vi "ProstateGetData.vi"() -> ()   [LabVIEW 2022 SP3]
uses:
  <instrlib>/vi.lib/Platform/portaccess.llb/Out Port8.vi
  <vilib>/DAQmx/create/channels.llb/DAQmx Create Channel (CO-Pulse Generation-Time).vi
  <resource>/objmgr/daqmx.rc
  <vilib>/DAQmx/configure/trigger.llb/DAQmx Start Trigger (Digital Edge).vi
  ScanningControl/Motion Controllers/-MotionRoutines/MotionGlobals.vi
  ScanningControl/Digitizers/-DigitizerRoutines/Digitizer.ctl
  ViewData/-ReadEye/ScaleMethod.ctl
  ScanningControl/Digitizers/-DigitizerRoutines/DigitizerID.ctl
  ScanningControl/Digitizers/-DigitizerRoutines/DigitizerSettings.ctl
  ScanningControl/Digitizers/-DigitizerRoutines/DigConfig.ctl
  C:/Windows/System32/ADQAPI_dotNet_helper.dll
panel:
  out "Digitizer Settings":T1={"Digitizer delay (us) "=0.0, "rf points per line"=2048, "lines per plane"=128, "Samp Rate (Hz)"=100000000.0, "Additional dig delay (us)"=0.0, "Voltage Scale"=0.4, "Pre-Looks"=0, "Offset delay (us)"=0.0, "bits A/D"=8, "Avg Num"=1, "DigTimeOut"=5.0, "Rel Dig Delay"=0.0, "Dig Ch"=0, "LeCroyCluster"={"LeCroy Channels"=[TRUE, FALSE, FALSE, FALSE], "LC read pt offset"=0.0, "Sweep Avg"=FALSE}, "Main Digitizer"=enum."NI Digitizer", "Dig Config"=enum."Single channel", "Digitizer ID Cluster"={"Acqiris/Alazar/SP ID"=[], "NI Instr Handles"=[], "LeCroy VISA"="", "GaGe Handle"={"Handle"=0, "Sample size"=0, "Resolution"=0, "Offset"=0, "Channels"=0, "Boards"=0}, "ATS Ref"="ATS9350", "Acqiris Address"=["PCI::INSTR0"], "ADQRef"=refnum, "adq_cu_ptr"=refnum}, "Trigger Settings"={"Trig Source"=1, "Trig Coupling"=0, "Trig Slope"=0, "Level (mV)"=1500.0}, "Bulk Acq"=FALSE, "Bulk Start Indexes"=[], "Data Ref RF"=refnum, "NI ID/Channel"=[], "Total Dig CH"=5, "Xtra Ann Trig delay (us)"=10.0, "Fix Z Delay?"=FALSE, "One Way Transmission?"=FALSE, "Data Ref Log"=refnum} {"Trigger Settings"."Trig Slope" items=["Positive", "Negative"]; "Trigger Settings"."Level (mV)" format="%.2f"; "Trigger Settings"."Trig Coupling" items=["DC 1 MOhm", "AC 1 MOhm", "DC 50 Ohm", "AC 50 Ohm"]; "Trigger Settings"."Trig Source" items=["Chan 1", "External"]; "Rel Dig Delay" format="%.2f"; "DigTimeOut" format="%.2f"; "Avg Num" min=1; "Offset delay (us)" format="%.2f"; "Additional dig delay (us)" format="%.2f"; "Digitizer delay (us)" format="%.2f"}
  in  "Digitizer Settings":T1={"Digitizer delay (us) "=0.0, "rf points per line"=2048, "lines per plane"=128, "Samp Rate (Hz)"=100000000.0, "Additional dig delay (us)"=0.0, "Voltage Scale"=0.4, "Pre-Looks"=0, "Offset delay (us)"=0.0, "bits A/D"=8, "Avg Num"=1, "DigTimeOut"=5.0, "Rel Dig Delay"=0.0, "Dig Ch"=0, "LeCroyCluster"={"LeCroy Channels"=[TRUE, FALSE, FALSE, FALSE], "LC read pt offset"=0.0, "Sweep Avg"=FALSE}, "Main Digitizer"=enum."NI Digitizer", "Dig Config"=enum."Single channel", "Digitizer ID Cluster"={"Acqiris/Alazar/SP ID"=[], "NI Instr Handles"=[], "LeCroy VISA"="", "GaGe Handle"={"Handle"=0, "Sample size"=0, "Resolution"=0, "Offset"=0, "Channels"=0, "Boards"=0}, "ATS Ref"="ATS9350", "Acqiris Address"=["PCI::INSTR0"], "ADQRef"=refnum, "adq_cu_ptr"=refnum}, "Trigger Settings"={"Trig Source"=1, "Trig Coupling"=0, "Trig Slope"=0, "Level (mV)"=1500.0}, "Bulk Acq"=FALSE, "Bulk Start Indexes"=[], "Data Ref RF"=refnum, "NI ID/Channel"=[], "Total Dig CH"=5, "Xtra Ann Trig delay (us)"=10.0, "Fix Z Delay?"=FALSE, "One Way Transmission?"=FALSE, "Data Ref Log"=refnum} {"Trigger Settings"."Trig Slope" items=["Positive", "Negative"]; "Trigger Settings"."Level (mV)" format="%.2f"; "Trigger Settings"."Trig Coupling" items=["DC 1 MOhm", "AC 1 MOhm", "DC 50 Ohm", "AC 50 Ohm"]; "Trigger Settings"."Trig Source" items=["Chan 1", "External"]; "Rel Dig Delay" format="%.2f"; "DigTimeOut" format="%.2f"; "Avg Num" min=1; "Offset delay (us)" format="%.2f"; "Additional dig delay (us)" format="%.2f"; "Digitizer delay (us)" format="%.2f"}
  in  "Attenuation":u8(slide) max=63 scale=0.0..63.0
  in  "File Name":string="name here"
  in  "GaGe":enum16{"CS1250", "CS8289"}(ring)=enum."CS8289"
  in  "Display mode":T5=enum."dB Scale"
  in  "Type of Mean":u16(ring) items=["Mean from lines", "Mean just lines", "Poly Mean", "No mean", "Filter"]
  in  "Volt Scale\n(Vpp)":i16(ring)=5
  in  "Frame #":i32
  in  "Hawk Noise":bool
  in  "Divide By":u8=1 min=1
  in  "Vecchio Hitachi?":bool=TRUE
  out "Frames":i8
  in  "Multiframe?":bool
  in  "hide ftp option?":bool=TRUE
  in  "location":u16(ring)=4 items=["VMMC", "U_HI", "Sloan Kett", "Columbia", "RRI Test", "St. Lukes"]
  in  "Probe":u16(ring) items=["Hitachi-fast (Vx3W)", "Hitachi-detailed (Vx3W)", "Hit U533 Ang5 Trans", "Hit U533 Ang4 Trans", "Hit U533 Ang3 Trans", "Hit U533 Ang6 Sag", "B&K 3535 with TGC", "B&K 3535 with no TGC", "B&K Hawk 8808 (S)", "B&K Hawk 8808 (T)", "B&K Hawk 8808 (Split)", "B&K Hawk 8658 (S)", "B&K Hawk 8658 (T)", "B&K Hawk 8663"]
  in  "Cal (F)/Acq (T) Counters":bool=TRUE
  in  "Transducer ID":i32
  in  "Operator":string
  in  "Keep":bool=TRUE
  in  "Show Thumbs":bool
  in  "distance?":bool
  in  "Erase data":bool
  in  "Case temp":string
  in  "Scan to View":u16(ring)
  in  "save data?":bool
  out "Raw data":dbl[][](graph)
  out "Digitizer Error Message":string
  in  "Set Digitizer":bool
  in  "start scan":bool
  in  "ExitSendCmd":bool
  # "Choose appropriate probe. Enter desired fields in Patient Info box as well as Operator initials and Transducer ID. Acquire data by pushing either Take Scan or the F1 key.  If regions of red appear in image, choose lower value for Gage Sens. Previous scans can be viewed by selecting the pull down menu Scan to View. If you do not wish to save a scan, select the Discard option while the scan is displayed. Thumbnails of all scans can be viewed by selecting View Thumbnails. When ready to save all data, select Save All Data. Erase data with Clear All Data and change RRI ID before taking a new set of data. Select Done when finished with all data acquisition or with a patient."
  # "File Controls"
  # "Discard"
  # "© 2000-2014 Riverside Research Institute"
  # "Need to place FTP subVI back in program if need"
  # "Uses Vecchio method of starting frame acq by sending a TTL signal to the hitachi"
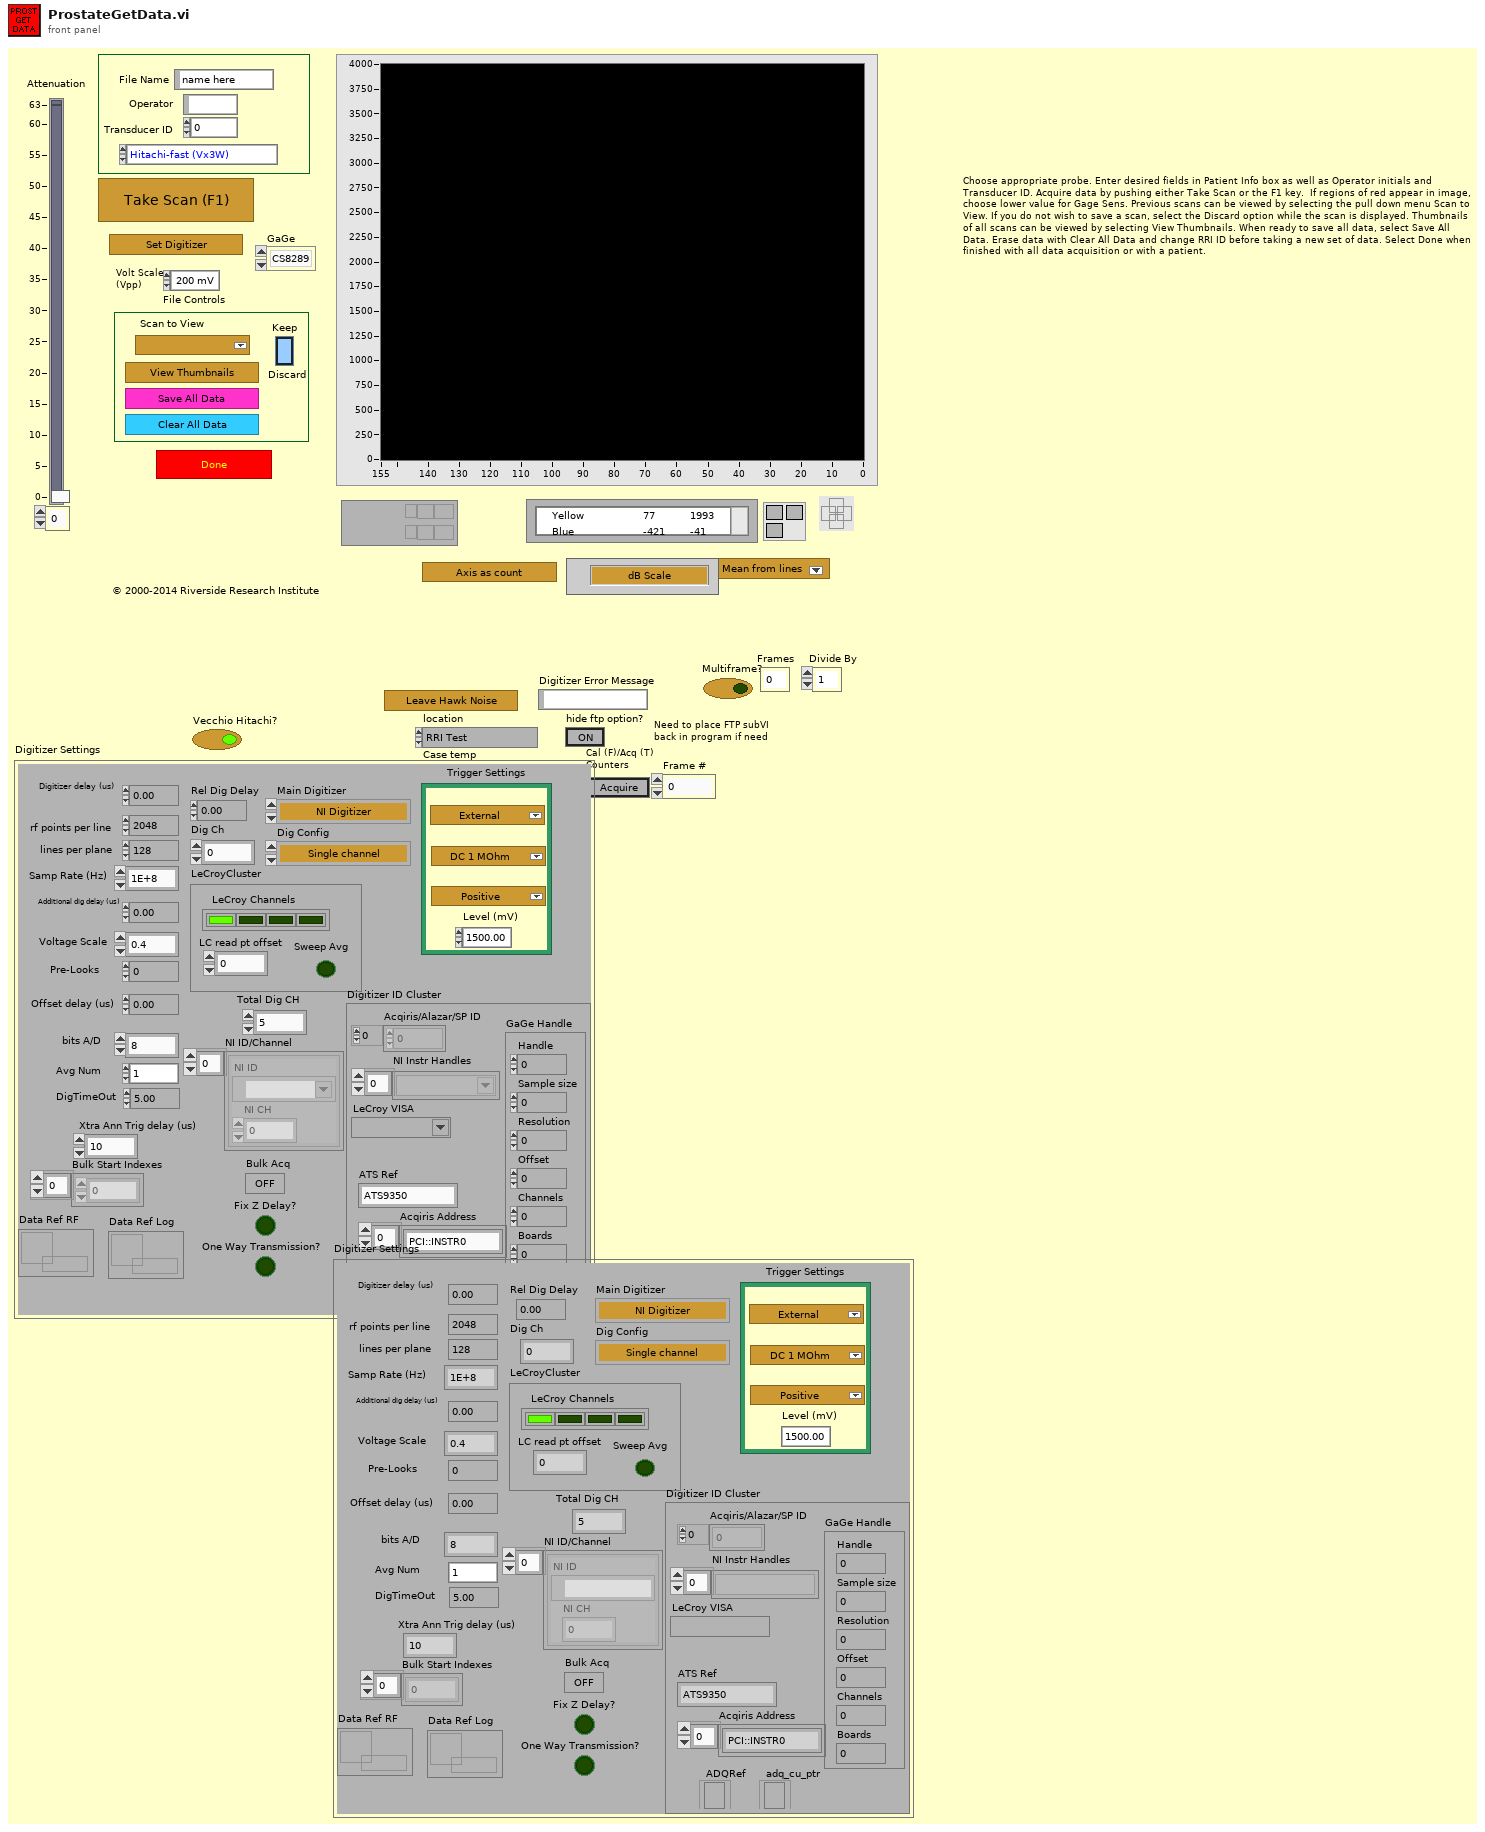
[diagram p1: front panel]
types:
  T1 = typedef "DigitizerSettings.ctl" = cluster{"Digitizer delay (us) ":dbl, "rf points per line":i32, "lines per plane":i32, "Samp Rate (Hz)":dbl, "Additional dig delay (us)":dbl, "Voltage Scale":dbl, "Pre-Looks":i32, "Offset delay (us)":dbl, "bits A/D":i8, "Avg Num":i32, "DigTimeOut":sgl, "Rel Dig Delay":sgl, "Dig Ch":i32, "LeCroyCluster":cluster{"LeCroy Channels":bool[], "LC read pt offset":dbl, "Sweep Avg":bool}, "Main Digitizer":T2, "Dig Config":T3, "Digitizer ID Cluster":T4, "Trigger Settings":cluster{"Trig Source":u16, "Trig Coupling":u16, "Trig Slope":u16, "Level (mV)":dbl}, "Bulk Acq":bool, "Bulk Start Indexes":i32[], "Data Ref RF":refnum<data-value>, "NI ID/Channel":cluster{"NI ID":refnum<k15>, "NI CH":i32}[], "Total Dig CH":i32, "Xtra Ann Trig delay (us)":dbl, "Fix Z Delay?":bool, "One Way Transmission?":bool, "Data Ref Log":refnum<data-value>}
  T2 = typedef "Digitizer.ctl" = enum16{"Acqiris Digitizer", "NI Digitizer", "LeCroy", "GaGe", "AlazarTech", "No Digitizer", "Teledyne"}
  T3 = typedef "DigConfig.ctl" = enum16{"Single channel", "2 Chans w/ 2 Acqiris", "2 Chans w/ 1 Acqiris", "5-CH Pulser New", "5-CH pulser w/ ann array", "5-pass style ann array", "Empty"}
  T4 = typedef "DigitizerID.ctl" = cluster{"Acqiris/Alazar/SP ID":u32[], "NI Instr Handles":refnum<k15>[], "LeCroy VISA":refnum<visa-resource-name>, "GaGe Handle":cluster{"Handle":u32, "Sample size":u32, "Resolution":i32, "Offset":i32, "Channels":u32, "Boards":u32}, "ATS Ref":string, "Acqiris Address":string[], "ADQRef":refnum<k24>, "adq_cu_ptr":refnum<k24>}
  T5 = typedef "ScaleMethod.ctl" = enum16{"Linear Abs Grey", "Log Grey Scale", "Linear Color Scale", "dB Scale", "Verasonics Doppler"}
  T6 = cluster{"RRI ID":string, "Hospital ID":string, "age":u16, "gender":string, "previously\nscanned":string, "PSA":sgl, "LOS":u8, "Ethnicty":u8, "Race":u8}
  T7 = cluster{"Handle":u32, "Sample size":u32, "Resolution":i32, "Offset":i32, "Channels":u32, "Boards":u32}
  T8 = typedef "MachineParams.ctl" = cluster{"machine type":enum16{"Hitachi", "B&K 3535", "B&K Hawk"}, "Number of frames":dbl, "Output Element":cluster{"Acquisition":cluster{"Sample Rate":dbl, "Clock Mode":enum16{"Internal", "External", "Reference"}, "Mode":string, "Depth":dbl, "Segment Size":dbl, "Trigger Timeout":dbl, "Trigger Holdoff":dbl, "Trigger Delay":dbl}, "V scale":cluster{"Voltage Scale":i16, "Offset":dbl, "Coupling":u16}, "Trigger":cluster{"Source":u16, "Coupling":u16, "Slope":u16, "Level":dbl}, "Vector Trigger Line":i16, "Total Delay (ms)":dbl, "Segment Count":u32, "lines per scan":i32}, "Thumb Size":cluster{"pixels in x":i16, "pixels in y":i16}, "Scan Info":cluster{"delay":sgl, "pivot distance":sgl, "sector scan angle":sgl, "operator":string, "Scan Mode":string, "location":string}}
  T9 = cluster{"acct":string, "passwrd":string, "ftp site":string, "subject":string, "file path":string, "recipients":string[], "SMTP Server":string}
  T10 = cluster{"Cal (F)/Acq (T) Counters":bool, "machine type":enum16{"Hitachi", "B&K 3535", "B&K Hawk"}}
  T11 = cluster{"Acquisition":cluster{"Sample Rate":dbl, "Clock Mode":enum16{"Internal", "External", "Reference"}, "Mode":string, "Depth":dbl, "Segment Size":dbl, "Trigger Timeout":dbl, "Trigger Holdoff":dbl, "Trigger Delay":dbl}, "V scale":cluster{"Voltage Scale":i16, "Offset":dbl, "Coupling":u16}, "Trigger":cluster{"Source":u16, "Coupling":u16, "Slope":u16, "Level":dbl}, "Vector Trigger Line":i16, "Total Delay (ms)":dbl, "Segment Count":u32, "lines per scan":i32}
  T12 = typedef "Header.ctl" = cluster{"header info":cluster{"Header":string, "Head length":i16}, "A/D info":cluster{"# rf points per line":u16, "# lines per scan":u16, "sample rate MHz":u16, "# A/D bits":i16, "# bytes per A/D":u16, "TGC Flag":u16, "A/D Type":string}, "Tranducer Info":cluster{"bandwidth":sgl, "center freq":sgl, "start freq":sgl, "ID":i32}, "Scan Info":cluster{"delay":sgl, "pivot distance":sgl, "sector scan angle":sgl, "operator":string, "Scan Mode":string, "location":string}, "Time/Date Info":cluster{"date":string, "time":string}, "RF Info":cluster{"RF file name":string, "RF file att":string, "RF cal file name":string, "RF cal file att":string}, "Patient Info":cluster{"ID":string, "extended ID":string, "age":u16, "sex":string, "previously\nscanned":string, "PSA":sgl, "LOS":u8, "Ethnicty 2":u8, "Race":u8}, "Tissue Type":cluster{"organ":i16, "disease type":i16, "disease location":i16, "IQ_pts":u16, "RcvBuffer":u8, "RcvFrame":u16, "IQBuff":u8, "IQFrame":u16, "IQPage":u8}, "Votage scaling":cluster{"Digitizer (dB)":sgl, "Gain (dB)":sgl, "Atten (dB)":sgl}, "Comment":string, "Misc Info":cluster{"avg num":u16, "c speed":i16, "Div By or SF zones":i16, "XMIT CHS":u8, "RCV CHS":u8, "Xmit angle":sgl}, "Therapy Parameters":cluster{"Theraputic Freq (MHz)":sgl, "Time on (s)":sgl, "Therapy amplitude (mV)":sgl, "Lines Before":u16, "Lines After":u16}, "Scan Settings":cluster{"Energy (uJ or V)":u8, "Damp (Ohm) or Fc":u8, "HP Filt (KHz)":u8, "LP Filt (MHz)":u8, "Gain (db)":u8, "prf (kHz)":sgl, "Distance between\nscan lines (um)":u16, "Distance between\nscan planes (um)":u16, "Scan line gap (um)":sgl, "Scan plane gap (um)":sgl}, "Compression Parameters":cluster{"F1 (MHz)":sgl, "F2 (MHz)":sgl, "% taper":sgl, "duration":sgl}, "Patient Info Xtra":cluster{"First Name":string, "Last Name":string, "Notes":string}, "ROI Box":u16[]}
  T13 = cluster{"File Name":string, "Keep?":bool, "Synth Foc?":bool}
  T14 = cluster{"File Name":string, "Keep?":bool, "Synth Foc?":bool}[]
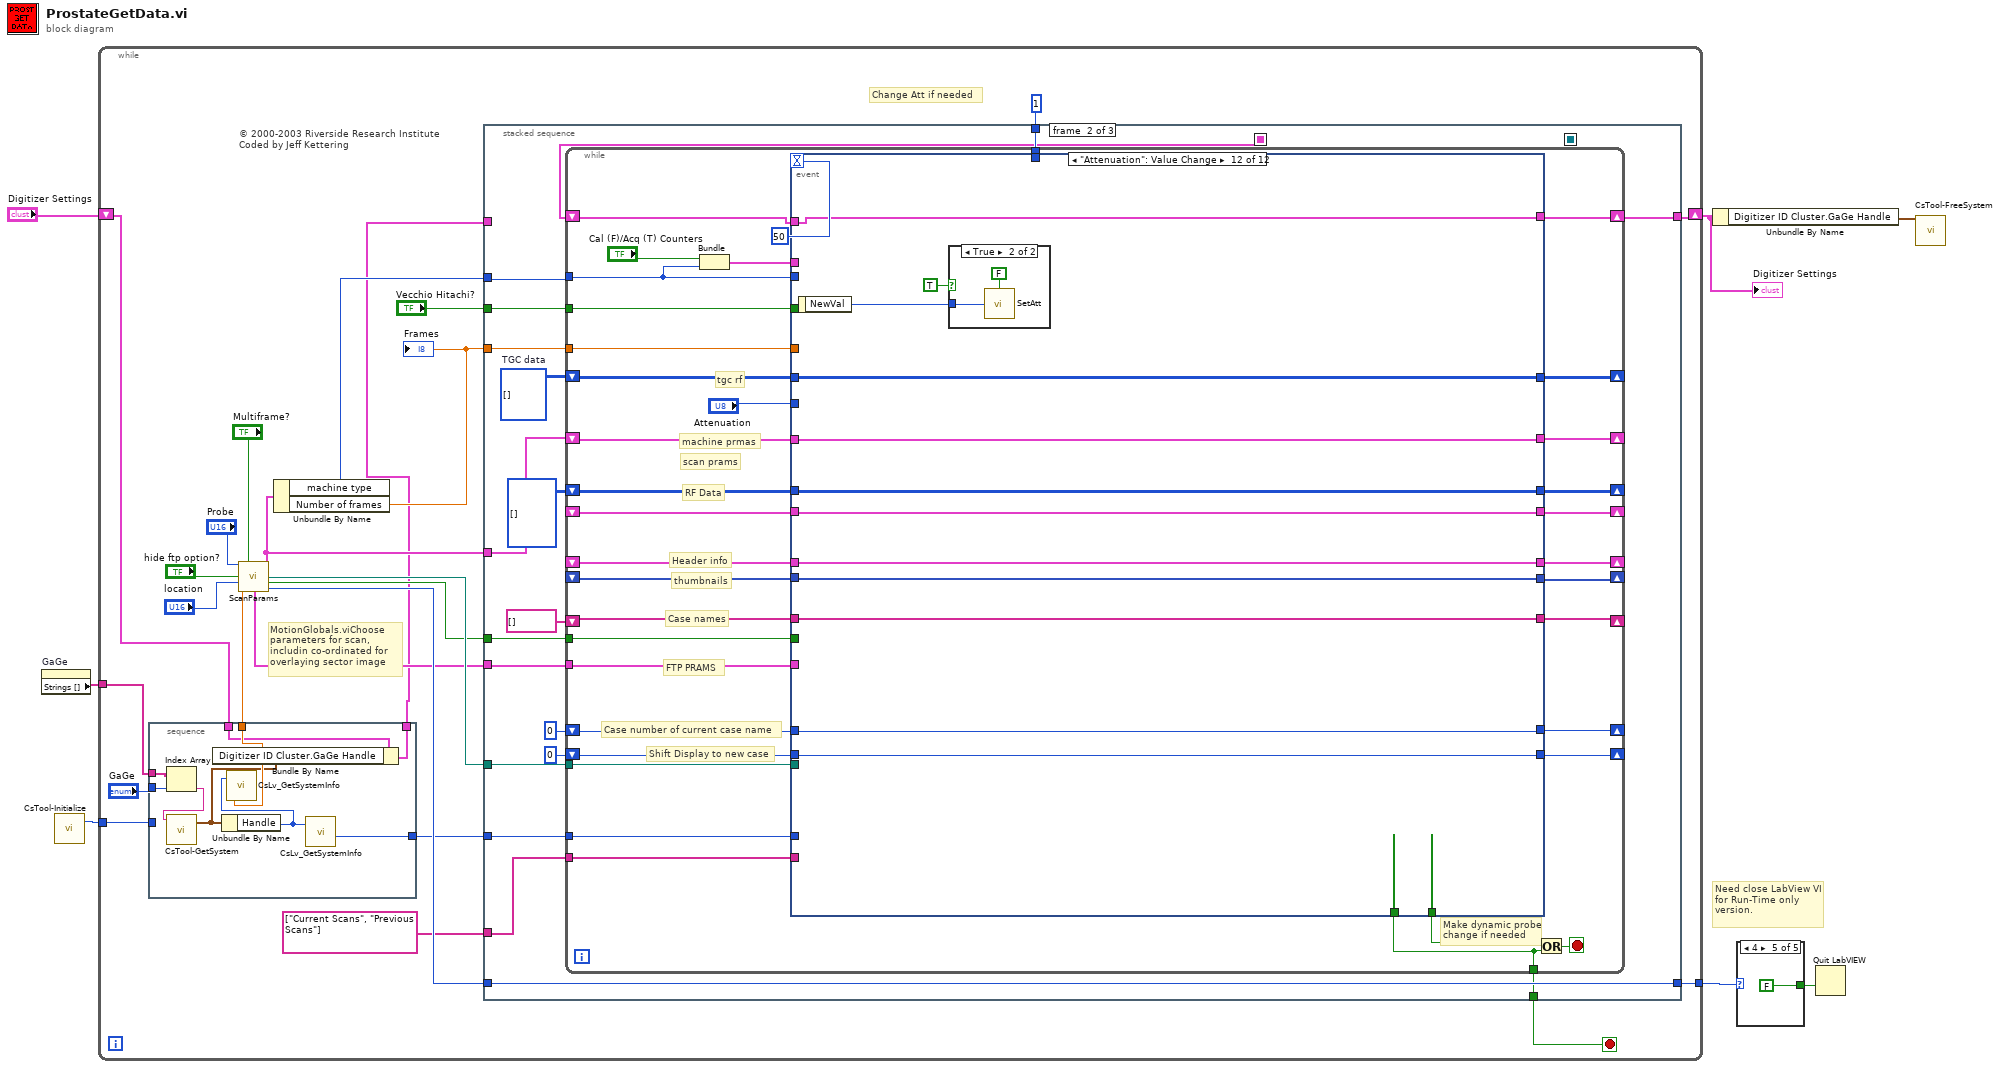
[diagram p0: block diagram]
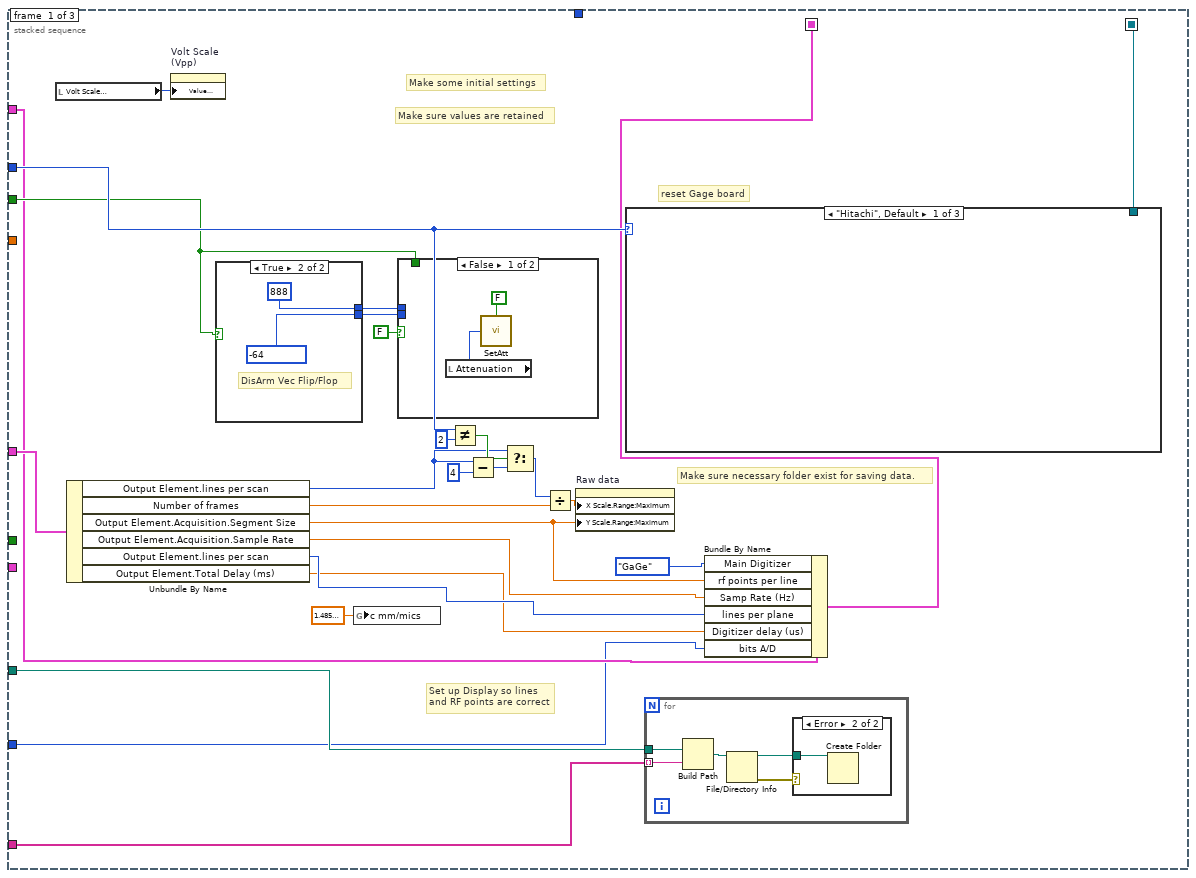
[diagram p2: hidden frame]
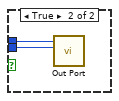
[diagram p3: hidden frame]
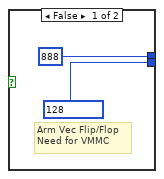
[diagram p5: hidden frame]
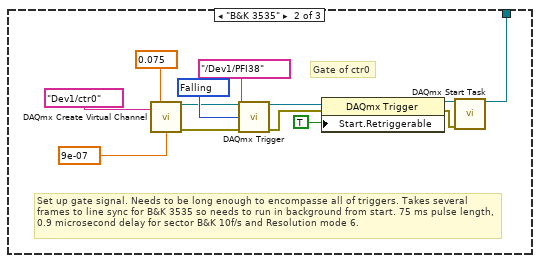
[diagram p6: hidden frame]
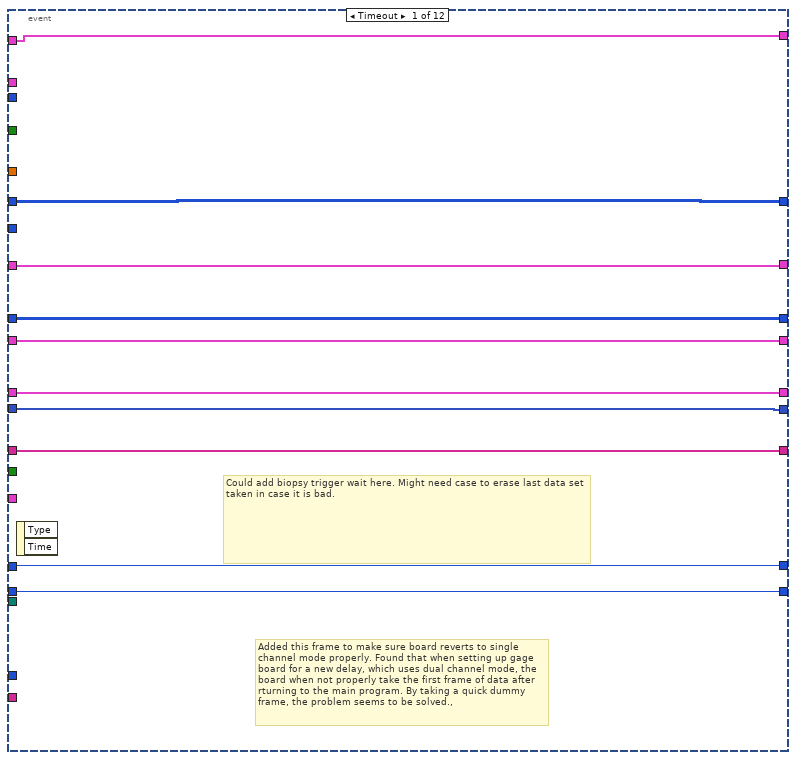
[diagram p8: hidden frame]
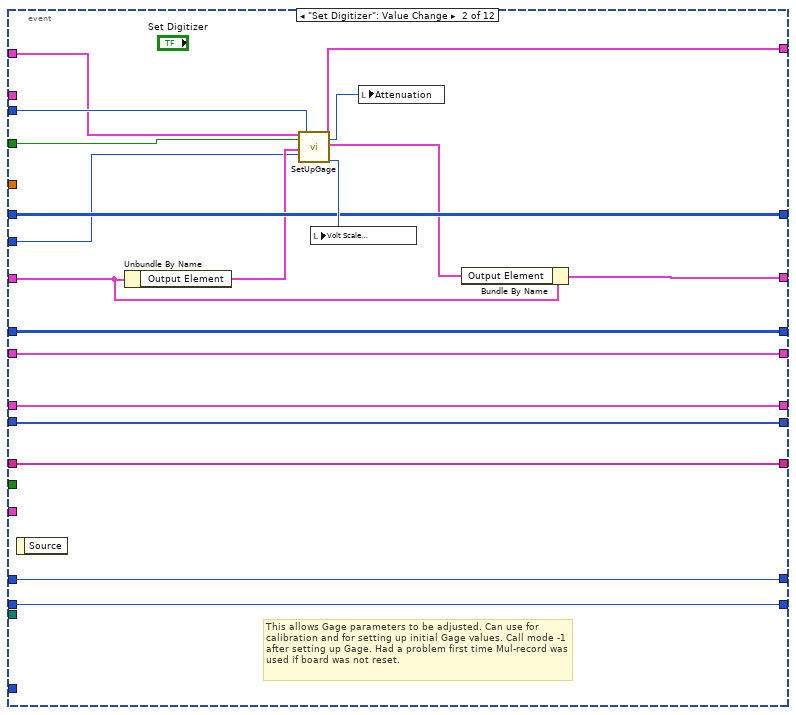
[diagram p9: hidden frame]
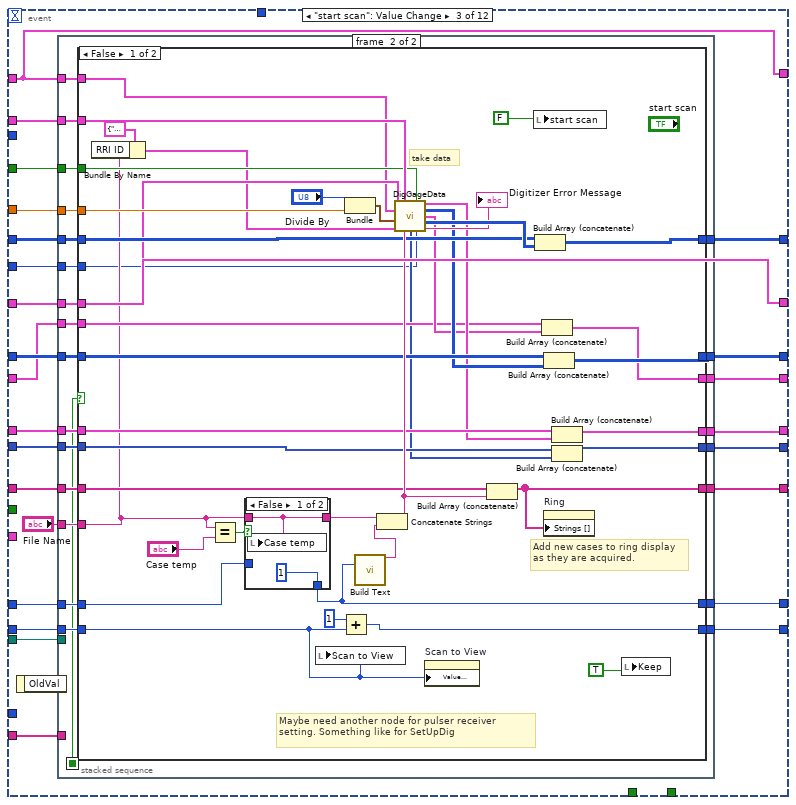
[diagram p10: hidden frame]
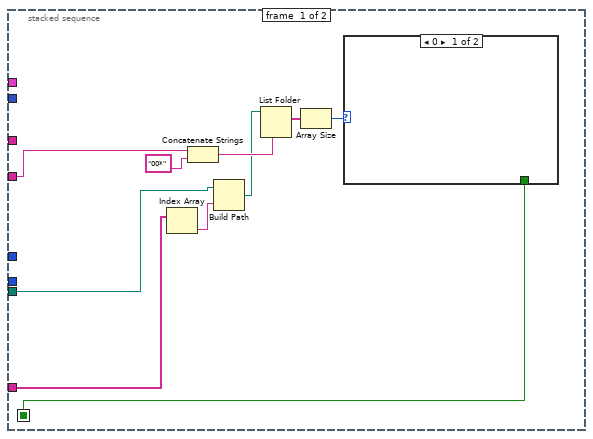
[diagram p11: hidden frame]
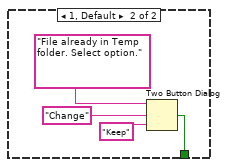
[diagram p12: hidden frame]
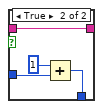
[diagram p13: hidden frame]
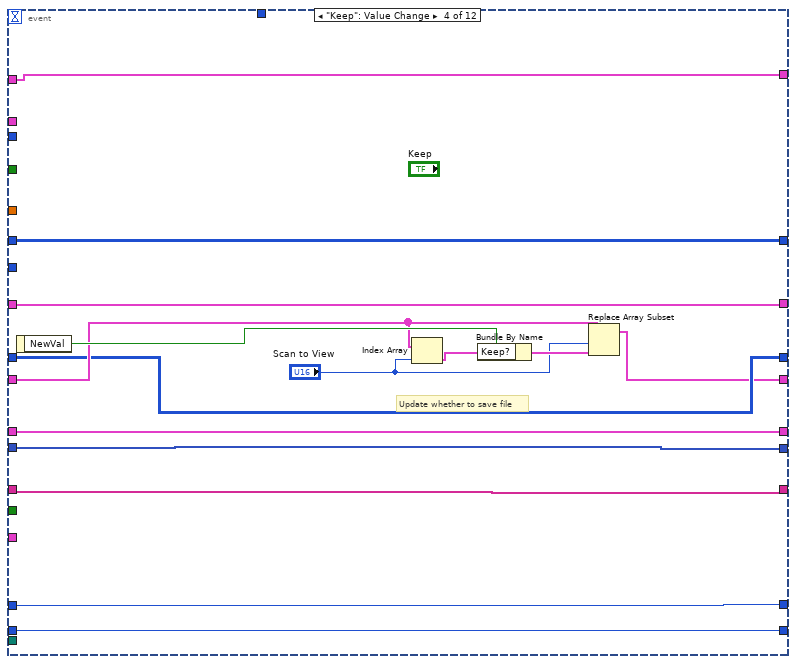
[diagram p15: hidden frame]
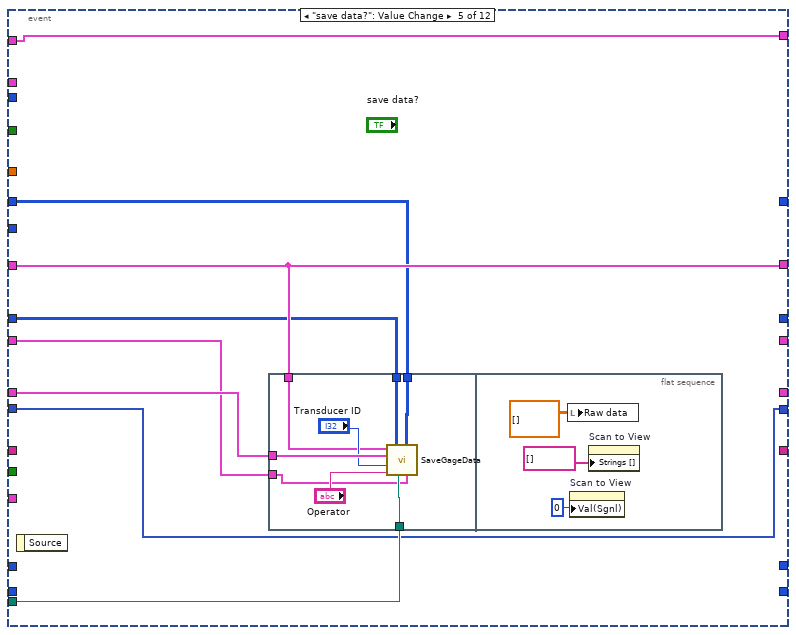
[diagram p16: hidden frame]
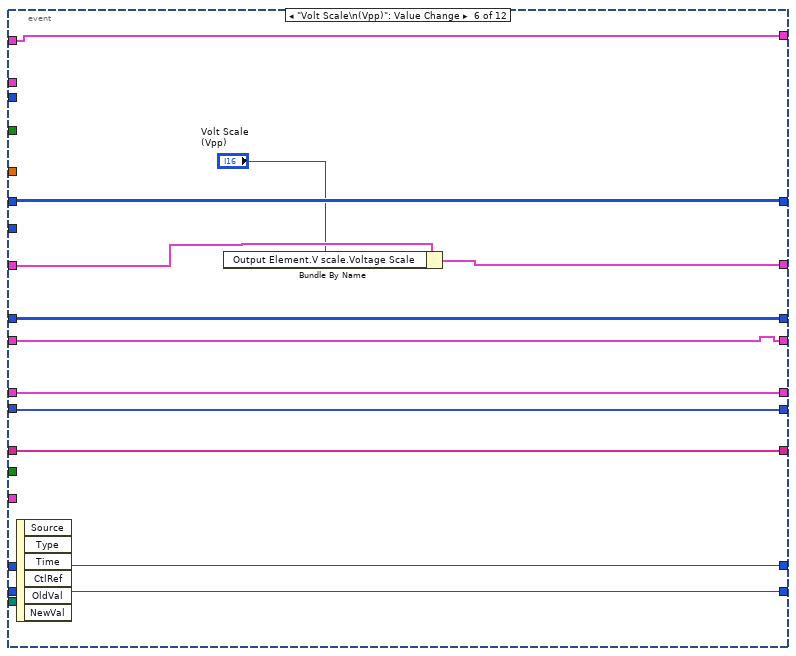
[diagram p17: hidden frame]
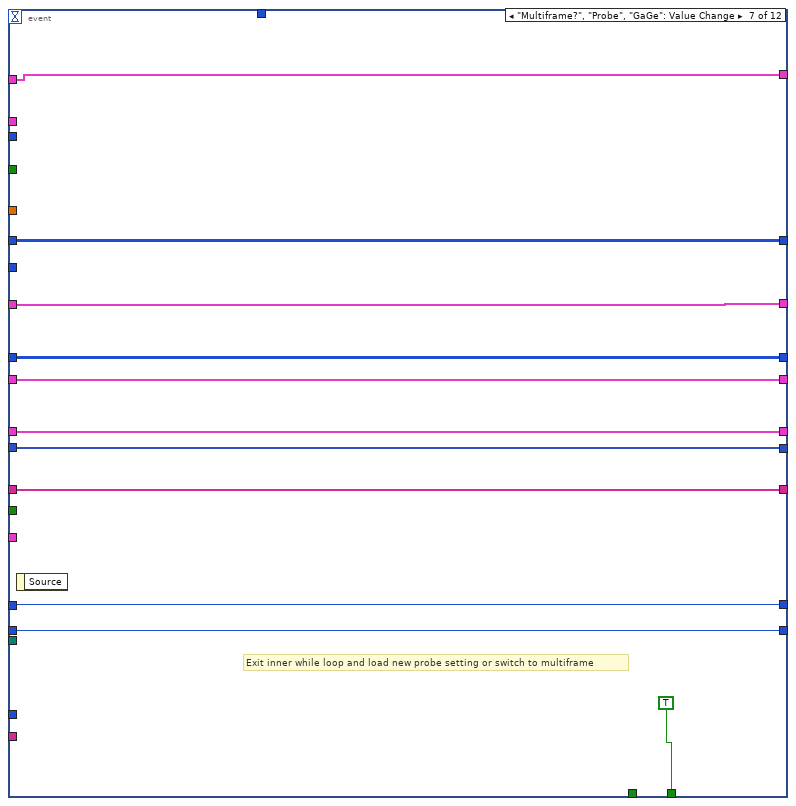
[diagram p18: hidden frame]
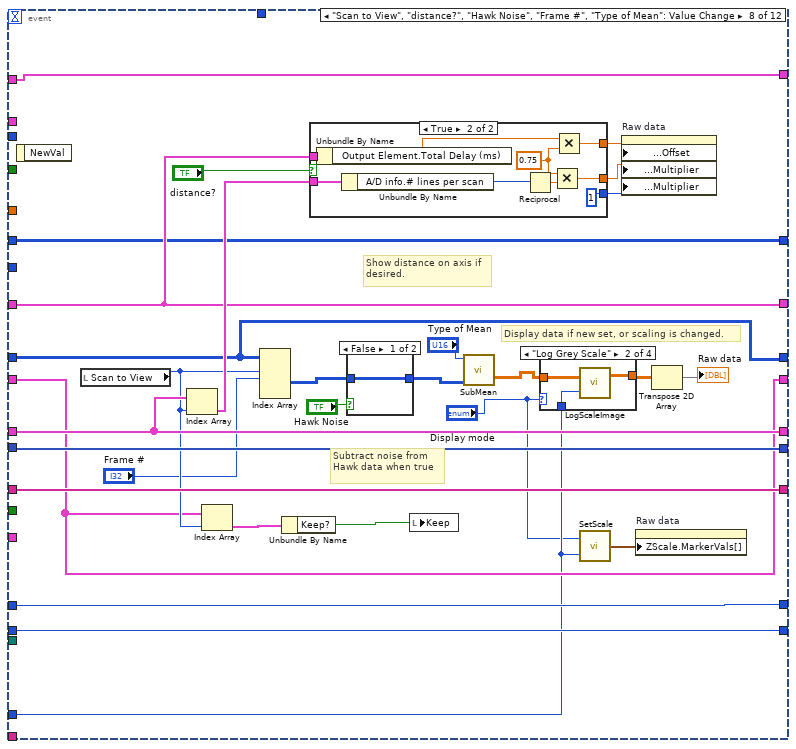
[diagram p19: hidden frame]
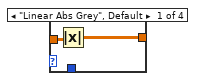
[diagram p20: hidden frame]
diagram:
  # "Need close LabView VI for Run-Time only version."
  n1 = property on="GaGe" class="Enum (strict)"() -> ("Strings []"=w5:string[])  [unwired: 2 in, 2 out]
  n2 = call <userlib>:"CsTool-Initialize.vi"() -> ("Number Of Systems"=w4:i32)  [unwired: 1 out]
  n3 = while {
    tunnel: [w30] -> w7
    tunnel: w5 -> [w14]
    tunnel: w4 -> [w12]
    shift-right: [w8] -> w1
    shift-left: "Digitizer Settings" -> [w10]
    stop <- w23 stop-if-true
    # "Change Att if needed"
    # "MotionGlobals.viChoose parameters for scan, includin co-ordinated for overlaying sector image"
    # "© 2000-2003 Riverside Research Institute\nCoded by Jeff Kettering"
    n4 = stacked-sequence {
      tunnel: [w40] -> w16
      tunnel: [w38] -> w17
      tunnel: w14 -> [w37]
      tunnel: "GaGe" -> [w35]
      tunnel: w12 -> [_]
      tunnel: w10 -> [w34]
      tunnel: [w32] -> w9
      frame #0 {
        n5 = Index Array(array=w37, index=w35) -> (element=w36:string)
        n6 = call <userlib>:"CsTool-GetSystem.vi"("Board Name (Any)"=w36) -> ("Handle Cluster"=w33:T7)  [unwired: 3 in, 1 out]
        n7 = Bundle By Name(cluster=w34, "Digitizer ID Cluster.GaGe Handle"=w33) -> (w32:T1)
        n8 = Unbundle By Name(w33) -> ("Handle"=w39:u32)
        n9 = call <userlib>:"CsLv_GetSystemInfo.vi"("Handle"=w39) -> ("Memory Size"=w38:dbl)  [unwired: 6 out]
        n10 = call <userlib>:"CsLv_GetSystemInfo.vi"("Handle"=w39) -> ("Sample Bits"=w40:u32)  [unwired: 6 out]
      }
    }
    n11 = call "ScanParams.vi"("Probe"="Probe", "Multiframes?"="Multiframe?", "hide ftp option? in"="hide ftp option?", "location in"="location", "GaGe Mem"=w17) -> ("Machine Params"=w15:T8, "directory to save data out"=w28:path, "hide ftp option? out"=w18:bool, "FTP params"=w19:T9, "location out"=w27:u16)  [unwired: 6 out]
    n12 = Unbundle By Name(w15) -> ("machine type"=w29:enum16{"Hitachi", "B&K 3535", "B&K Hawk"}, "Number of frames"=w22:dbl)
    "Frames" <- w22
    n13 = stacked-sequence {
      seq-local: [w53 _ _] -> [_ _ w480]
      seq-local: [w41 _ _] -> [_ w95 _]
      tunnel: w29 -> [w58 w113 w481]
      tunnel: 1 -> [_ w112 _]
      tunnel: w28 -> [w67 w110 _]
      tunnel: w27 -> [_ w108 _]
      tunnel: w22 -> [_ w109 _]
      tunnel: [_ w108 _] -> w30
      tunnel: w15 -> [w64 w103 _]
      tunnel: [_ w104 _] -> w23
      tunnel: "Vecchio Hitachi?" -> [w50 w107 _]
      tunnel: w19 -> [_ w106 _]
      tunnel: w18 -> [_ w105 _]
      tunnel: w16 -> [w42 w98 _]
      tunnel: string[] ["Current Scans", "Previous Scans"] -> [w49 w97 _]
      tunnel: w9 -> [w48 _ _]
      tunnel: [_ w96 _] -> w8
      frame #0 {
        # "Make sure values are retained"
        # "Set up Display so lines and RF points are correct"
        # "Make sure necessary folder exist for saving data."
        # "reset Gage board"
        # "Make some initial settings"
        n14 = local read "Volt Scale\n(Vpp)"() -> (w54:i16)
        n15 = Unbundle By Name(w64) -> ("Output Element.lines per scan"=w57:i32, "Number of frames"=w65:dbl, "Output Element.Acquisition.Segment Size"=w46:dbl, "Output Element.Acquisition.Sample Rate"=w47:dbl, "Output Element.lines per scan"=w45:i32, "Output Element.Total Delay (ms)"=w44:dbl)
        n16 = property on="Volt Scale\n(Vpp)" class="Ring (strict)"("Value (Signaling)"=w54) -> ()  [unwired: 2 in, 2 out]
        n17 = case shown="True" w50 {
          tunnel: [u32 888 ("Port Address") u32 888 ("Port Address")] -> w56
          tunnel: [u8 128 i8 -64] -> w55
          frame False {
            # "Arm Vec Flip/Flop\nNeed for VMMC"
          }
          frame True {
            # "DisArm Vec Flip/Flop"
          }
        }
        n18 = global write "MotionGlobals.vi" "c mm/mics"(sgl 1.485 ("c mm/mics")) -> ()
        n19 = case shown="False" FALSE {
          tunnel: w56 -> [_ w71]
          tunnel: w55 -> [_ w70]
          tunnel: w50 -> [_ _]
          frame False {
            n20 = local read "Attenuation"() -> (w68:u8)
            n21 = call "SetAtt.vi"("Arm Trigs?"=FALSE, "Attenuation"=w68) -> ()  [unwired: 4 in]
          }
          frame True {
            n22 = call-poly <instrlib>:"Out Port.vi"("write value"=w70, "address"=w71) -> ()  [unwired: 1 in, 7 out]
          }
        }
        n23 = Not Equal?(x=w58, y=2) -> (x != y?=w62:bool)
        n24 = Subtract(x=w57, y=4) -> (x-y=w60:i32)
        n25 = Select(t=w57, s=w62, f=w60) -> (s? t:f=w59:i32)
        n26 = Divide(x=w59, y=w65) -> (x/y=w66:dbl)
        n27 = property on="Raw data" class="IntGraph (strict)"("X Scale.Range:Maximum"=w66, "Y Scale.Range:Maximum"=w46) -> ()  [unwired: 2 in, 2 out]
        n28 = case shown="\"Hitachi\", Default" w58 {
          tunnel: [_ w94 _] -> w53
          frame "Hitachi", Default {
          }
          frame "B&K 3535" {
            w91 = 10171 items=["Rising"=10280, "Falling"=10171] ("edge")
            # "Gate of ctr0"
            # "Set up gate signal. Needs to be long enough to encompasse all of triggers. Takes several frames to line sync for B&K 3535 so needs to run in background from start. 75 ms pulse length, 0.9 microsecond delay for sector B&K 10f/s and Resolution mode 6."
            n29 = call-poly <vilib>:"DAQmx Create Virtual Channel.vi"("high time"=0.075 ("pulse width (s or cycles)"), "counter"=tag "Dev1/ctr0", "initial delay"=9e-07 ("pulse width (s or cycles)")) -> ("task out"=w89:refnum<k21>, "error out"=w90:errorcluster)  [unwired: 6 in, 5 out]
            n30 = call-poly <vilib>:"DAQmx Trigger.vi"("task/channels in"=w89, "source"=tag "/Dev1/PFI38", "edge"=w91, "error in"=w90) -> ("task out"=w86:refnum<k21>, "error out"=w87:errorcluster)  [unwired: 10 out]
            n31 = property class="DAQmx Trigger"(reference=w86, error in=w87, "Start.Retriggerable"=TRUE) -> (reference out=w92:refnum<k21>, error out=w93:errorcluster)
            n32 = call <vilib>:"DAQmx Start Task.vi"("task/channels in"=w92, "error in"=w93) -> ("task out"=w94:refnum<k21>)  [unwired: 13 out]
          }
          frame "B&K Hawk" {
          }
        }
        n33 = for {
          tunnel: w67 -> [w75]
          tunnel: w49 -> [w72] mode=indexing
          n34 = Build Path(base path=w75, name or relative path=w72) -> (appended path=w76:path)
          n35 = File/Directory Info(path=w76) -> (path out=w73:path, error out=w74:errorcluster)  [unwired: 1 in, 5 out]
          n36 = case shown="Error" w74 {
            tunnel: w73 -> [_ w77]
            frame No Error {
            }
            frame Error {
              n37 = Create Folder(path (use dialog)=w77) -> ()  [unwired: 1 in, 4 out]
            }
          }
        }
        n38 = Bundle By Name(cluster=w48, "Main Digitizer"=Digitizer."GaGe", "rf points per line"=w46, "Samp Rate (Hz)"=w47, "lines per plane"=w45, "Digitizer delay (us)"=w44, "bits A/D"=w42) -> (w41:T1)
      }
      frame #1 {
        w111 = i16[][][] []  # TGC data
        n39 = while {
          tunnel: w109 -> [w140]
          tunnel: w110 -> [w138]
          shift-left: w111 -> [w141]
          shift-right: [w127] -> _
          tunnel: w112 -> [w142]
          shift-left: w103 -> [w144]
          shift-right: [w143] -> _
          tunnel: w113 -> [w130]
          shift-left: _ -> [w145]
          shift-right: [w124] -> _
          shift-left: 0 -> [w146]
          shift-right: [w121] -> _
          shift-left: string[] [] ("Array Constant") -> [w147]
          shift-right: [w123] -> _
          shift-left: 0 -> [w148]
          shift-right: [w122] -> _
          shift-left: _ -> [w149]
          shift-right: [w125] -> _
          tunnel: w107 -> [w137]
          shift-right: [w126] -> _
          shift-left: i16[][][][] [] -> [w136]
          tunnel: w106 -> [w135]
          tunnel: w105 -> [w134]
          tunnel: [w132] -> w104
          shift-right: [w120] -> _
          shift-left: _ -> [w119]
          tunnel: w98 -> [w118]
          tunnel: w97 -> [w117]
          shift-right: [w114] -> w96
          shift-left: w95 -> [w115]
          stop <- w139 stop-if-true
          # "Header info"
          # "RF Data"
          # "machine prmas"
          # "Shift Display to new case"
          # "Case number of current case name"
          # "FTP PRAMS"
          # "scan prams"
          # "tgc rf"
          # "thumbnails"
          # "Case names"
          # "Make dynamic probe change if needed"
          n40 = Bundle("Cal (F)/Acq (T) Counters"="Cal (F)/Acq (T) Counters", "machine type"=w130) -> (w129:T10)  [unwired: 1 out]
          n41 = event shown="[11] \"Attenuation\": Value Change" {
            selector: _ -> [_ _ _ _ _ _ _ _ _ _ _ _]
            dyn-events: _ -> [_ _ _ _ _ _ _ _ _ _ _ _]
            timeout: 50 -> [_ _ _ _ _ _ _ _ _ _ _ _]
            tunnel: w145 -> [w153 w169 w199 w305 w313 w339 w347 w369 w413 w431 _ w473]
            tunnel: w136 -> [w154 w170 w194 w300 w315 w340 w346 w373 w414 w433 _ w472]
            tunnel: w138 -> [_ _ w182 _ w319 _ _ _ _ _ w457 _]
            tunnel: w149 -> [w158 w175 w200 w298 w317 w342 w351 w375 w416 w432 _ w470]
            tunnel: [_ _ _ _ _ _ _ _ _ _ w456 _] -> w132
            tunnel: w135 -> [_ _ _ _ _ _ _ _ _ _ w459 _]
            tunnel: w134 -> [_ _ _ _ _ _ _ _ _ _ w458 _]
            tunnel: [_ _ _ _ _ _ TRUE _ _ _ _ _] -> w133
            tunnel: w144 -> [w159 w165 w186 w307 w318 w334 w352 w376 w409 w436 _ w471]
            tunnel: w130 -> [_ w178 _ _ _ _ _ _ _ _ _ _]
            tunnel: w142 -> [_ _ _ _ _ _ _ _ _ _ _ _]
            tunnel: w137 -> [_ w177 w202 _ _ _ _ _ _ _ _ _]
            tunnel: [w159 w164 w186 w307 w318 w333 w352 w376 w409 w436 _ w471] -> w143
            tunnel: w129 -> [_ _ w203 _ _ _ _ _ _ _ _ _]
            tunnel: [w158 w175 w191 w298 _ w342 w351 w375 w416 w423 _ w470] -> w125
            tunnel: w141 -> [w152 w171 w201 w306 w316 w341 w345 w374 w415 w434 _ w475]
            tunnel: w148 -> [w156 w174 w198 w304 _ w337 w350 w372 w411 w429 _ w469]
            tunnel: w146 -> [w157 w173 w193 w303 _ w336 w349 w371 w410 w428 _ w468]
            tunnel: [w157 w173 w197 w303 _ w336 w349 w371 w410 w427 _ w468] -> w121
            tunnel: [w156 w174 w196 w304 _ w337 w350 w372 w411 w426 _ w469] -> w122
            tunnel: w147 -> [w155 w172 w195 w302 _ w338 w348 w370 w412 w430 _ w474]
            tunnel: [w155 w172 w192 w302 _ w338 w348 w370 w412 w425 _ w474] -> w123
            tunnel: [w154 w170 w190 w300 _ w340 w346 w373 w414 w422 _ w472] -> w126
            tunnel: [w152 w171 w189 w306 _ w341 w345 w374 w415 w421 _ w475] -> w127
            tunnel: [w153 w169 w188 w305 w313 w339 w347 w369 w413 w424 _ w473] -> w124
            tunnel: w140 -> [_ _ w187 _ _ _ _ _ _ _ _ _]
            tunnel: [w151 w168 w184 w299 _ w335 w344 w363 w406 w420 _ w467] -> w120
            tunnel: w119 -> [w151 w168 w185 w301 w314 w335 w344 w363 w406 w419 _ w467]
            tunnel: w118 -> [_ _ _ _ _ _ _ w357 _ _ _ _]
            tunnel: w117 -> [_ _ w181 _ _ _ _ _ _ _ _ _]
            tunnel: "Attenuation" -> [_ w162 w180 _ _ _ _ _ _ _ _ _]
            tunnel: w115 -> [w150 w161 w179 w297 w312 w331 w343 w354 w405 w418 w451 w466]
            tunnel: [w150 w160 w179 w297 w312 w331 w343 w354 w405 w418 w451 w466] -> w114
            event Timeout {
              # "Could add biopsy trigger wait here. Might need case to erase last data set taken in case it is bad."
              # "Added this frame to make sure board reverts to single channel mode properly. Found that when setting up gage board for a new delay, which uses dual channel mode, the board when not properly take the first frame of data after rturning to the main program. By taking a quick dummy frame, the problem seems to be solved.,"
              n42 = event-data() -> ()  [unwired: 3 out]
            }
            event "Set Digitizer": Value Change {
              # "This allows Gage parameters to be adjusted. Can use for calibration and for setting up initial Gage values. Call mode -1 after setting up Gage. Had a problem first time Mul-record was used if board was not reset."
              n43 = event-data() -> ()  [unwired: 2 out]
              n44 = Unbundle By Name(w165) -> ("Output Element"=w167:T11)
              n45 = call "SetUpGage.vi"("Digitizer Settings"=w161, "Vecchio Hitachi?"=w177, "Acquisition In"=w167, "Attenuation"=w162, "Machine Type"=w178) -> ("Digitizer Settings Out"=w160:T1, "Attenuation out"=w163:u8, "Acquisition Settings Out"=w166:T11, "Voltage Scale (pp) OUT"=w176:i16)  [unwired: 8 in, 3 out]
              n46 = local write "Volt Scale\n(Vpp)"(w176) -> ()
              n47 = local write "Attenuation"(w163) -> ()
              n48 = Bundle By Name(cluster=w165, "Output Element"=w166) -> (w164:T8)
            }
            event "start scan": Value Change {
              n49 = event-data() -> ()  [unwired: 2 out]
              n50 = stacked-sequence {
                seq-local: [w208 _] -> [_ w220]
                tunnel: w203 -> [_ w241]
                tunnel: w202 -> [_ w240]
                tunnel: w201 -> [_ w239]
                tunnel: w200 -> [_ w238]
                tunnel: w199 -> [_ w237]
                tunnel: w198 -> [_ w236]
                tunnel: [_ w235] -> w197
                tunnel: [_ w234] -> w196
                tunnel: w195 -> [_ w233]
                tunnel: w194 -> [_ w232]
                tunnel: w193 -> [_ w231]
                tunnel: [_ w230] -> w192
                tunnel: [_ w229] -> w191
                tunnel: [_ w228] -> w190
                tunnel: [_ w227] -> w189
                tunnel: [_ w226] -> w188
                tunnel: w187 -> [_ w225]
                tunnel: w186 -> [_ w224]
                tunnel: w185 -> [_ w223]
                tunnel: [_ w222] -> w184
                tunnel: "File Name" -> [w209 w221]
                tunnel: w182 -> [w205 _]
                tunnel: w181 -> [w207 _]
                tunnel: w180 -> [_ w219]
                tunnel: w179 -> [_ w218]
                frame #0 {
                  n51 = Index Array(array=w207) -> (element=w206:string)  [unwired: 1 in]
                  n52 = Concatenate Strings(w209, "00*") -> (w213:string)
                  n53 = Build Path(base path=w205, name or relative path=w206) -> (appended path=w204:path)
                  n54 = List Folder(path=w204, pattern=w213) -> (filenames=w212:string[])  [unwired: 1 in, 4 out]
                  n55 = Array Size(array=w212) -> (size(s)=w211:i32)
                  n56 = case shown="0" w211 {
                    tunnel: [_ w214] -> w208
                    frame 0 {
                    }
                    frame 1, Default {
                      n57 = Two Button Dialog(message="File already in Temp folder. Select option.", 1:"Keep" ("F button name (\"Cancel\")"), 2:"Change" ("T button name (\"OK\")")) -> (T button?=w214:bool)
                    }
                  }
                }
                frame #1 {
                  n58 = case shown="False" w220 {
                    tunnel: w241 -> [w276 _]
                    tunnel: w240 -> [w275 _]
                    tunnel: w239 -> [w274 w296]
                    tunnel: w238 -> [w273 w295]
                    tunnel: w237 -> [w272 w294]
                    tunnel: w236 -> [w271 w292]
                    tunnel: [w270 w291] -> w235
                    tunnel: [w245 w292] -> w234
                    tunnel: w233 -> [w269 w293]
                    tunnel: w232 -> [w268 w290]
                    tunnel: w231 -> [w266 w291]
                    tunnel: [w265 w293] -> w230
                    tunnel: [w264 w295] -> w229
                    tunnel: [w260 w290] -> w228
                    tunnel: [w259 w296] -> w227
                    tunnel: [w258 w294] -> w226
                    tunnel: w225 -> [w257 _]
                    tunnel: w224 -> [w254 _]
                    tunnel: w223 -> [w251 w289]
                    tunnel: [w250 w289] -> w222
                    tunnel: w221 -> [w246 _]
                    tunnel: w219 -> [w243 _]
                    tunnel: w218 -> [w242 _]
                    frame False {
                      # "Maybe need another node for pulser receiver setting. Something like for SetUpDig"
                      # "Add new cases to ring display\nas they are acquired."
                      # "take data"
                      n59 = Bundle By Name(cluster=T6 {"RRI ID"="abc", "Hospital ID"="aslkdjf", "age"=0, "gender"="M", "previously\nscanned"="N", "PSA"=0.0, "LOS"=2, "Ethnicty"=2, "Race"=6} ("Patient Info"), "RRI ID"=w246) -> (w249:T6)
                      n60 = Equal?(x=w246, y="Case temp") -> (x = y?=w282:bool)
                      n61 = case shown="False" w282 {
                        tunnel: w271 -> [_ w286]
                        tunnel: [1 w285] -> w245
                        tunnel: w246 -> [w283 w288]
                        tunnel: [w283 w288] -> w281
                        frame False {
                          n62 = local write "Case temp"(w283) -> ()
                        }
                        frame True {
                          n63 = Add(x=1, y=w286) -> (x+y=w285:i32)
                        }
                      }
                      n64 = local write "Scan to View"(w266) -> ()
                      n65 = Add(x=1, y=w266) -> (x+y=w270:i32)
                      n66 = Bundle("Divide By"="Divide By", "Number of frames"=w257) -> (w277:cluster{"Divide By":u8, "Number of frames":dbl})  [unwired: 1 out]
                      n67 = call "Build Text"("s"=w245) -> ("Result"=w244:string)  [unwired: 13 in, 1 out]
                      n68 = Concatenate Strings(w281, w244) -> (w279:string)
                      n69 = call "DigGageData.vi"("Machine Params"=w254, "Counter Params"=w276, "Vecchio Hitachi?"=w275, "Digitizer Settings"=w242, "Frame Prams"=w277, "Patient Info"=w249, "File Name"=w279, "Attenuation"=w243) -> ("output cluster"=w253:T12, "Data"=w255:i16[][][], "Scan Params"=w252:T13, "TGC data"=w278:i16[][], "Array"=w247:picture[], "Error Message"=→"Digitizer Error Message":string)  [unwired: 2 in]
                      n70 = property on="Scan to View" class="Ring (strict)"("Value (Signaling)"=w266) -> ()  [unwired: 2 in, 2 out]
                      n71 = Build Array (concatenate)(w269, w279) -> (w265:string[])
                      n72 = local write "start scan"(FALSE) -> ()
                      n73 = Build Array (concatenate)(w274, w278) -> (w259:i16[][][])
                      n74 = Build Array (concatenate)(w251, w252) -> (w250:T14)
                      n75 = Build Array (concatenate)(w268, w255) -> (w260:i16[][][][])
                      n76 = property on="Ring" class="Ring (strict)"("Strings []"=w265) -> ()  [unwired: 2 in, 2 out]
                      n77 = Build Array (concatenate)(w273, w253) -> (w264:T12[])
                      n78 = Build Array (concatenate)(w272, w247) -> (w258:picture[])
                      n79 = local write "Keep"(TRUE) -> ()
                    }
                    frame True {
                    }
                  }
                }
              }
            }
            event "Keep": Value Change {
              # "Update whether to save file"
              n80 = event-data() -> ("NewVal"=w309:bool)  [unwired: 1 out]
              n81 = Index Array(array=w301, index="Scan to View") -> (element=w311:T13)
              n82 = Bundle By Name(cluster=w311, "Keep?"=w309) -> (w310:T13)
              n83 = Replace Array Subset(array=w301, new element=w310, index="Scan to View") -> (w299:T14)
            }
            event "save data?": Value Change {
              n84 = event-data() -> ()  [unwired: 2 out]
              n85 = flat-sequence {
                tunnel: w317 -> [w327]
                tunnel: w319 -> [w326]
                tunnel: w315 -> [w322]
                tunnel: w318 -> [w323]
                tunnel: w316 -> [w321]
                tunnel: w314 -> [w320]
                frame #0 {
                  n86 = call "SaveGageData.vi"("Keep array"=w320, "TGC data"=w321, "folder path"=w326, "Data"=w322, "operator"="Operator", "ID"="Transducer ID", "Array"=w327, "Machine Params"=w323) -> ()  [unwired: 1 in, 3 out]
                }
                frame #1 {
                  n87 = local write "Raw data"(dbl[][] [] ("Raw data")) -> ()
                  n88 = property on="Scan to View" class="Ring (strict)"("Val(Sgnl)"=u16 0 ("Value (Signaling)")) -> ()  [unwired: 2 in, 2 out]
                  n89 = property on="Scan to View" class="Ring (strict)"("Strings []"=string[] []) -> ()  [unwired: 2 in, 2 out]
                }
              }
            }
            event "Volt Scale\n(Vpp)": Value Change {
              n90 = event-data() -> ()  [unwired: 7 out]
              n91 = Bundle By Name(cluster=w334, "Output Element.V scale.Voltage Scale"="Volt Scale\n(Vpp)") -> (w333:T8)
            }
            event "Multiframe?", "Probe", "GaGe": Value Change {
              # "Exit inner while loop and load new probe setting or switch to multiframe"
              n92 = event-data() -> ()  [unwired: 2 out]
            }
            event "Scan to View", "distance?", "Hawk Noise", "Frame #", "Type of Mean": Value Change {
              # "Subtract noise from Hawk data when true"
              # "Display data if new set, or scaling is changed."
              # "Show distance on axis if\ndesired."
              n93 = event-data() -> ()  [unwired: 2 out]
              n94 = local read "Scan to View"() -> (w364:u16)
              n95 = Index Array(array=w375, index=w364) -> (element=w381:T12)
              n96 = Index Array(array=w363, index=w364) -> (element=w362:T13)
              n97 = Index Array(array=w373, index (dim 0)=w364, index (dim 1)="Frame #") -> (element=w366:i16[][])  [unwired: 2 in]
              n98 = Unbundle By Name(w362) -> ("Keep?"=w382:bool)
              n99 = case shown="True" "distance?" {
                tunnel: [0 w402] -> w379
                tunnel: [w394 w401] -> w378
                tunnel: [w394 1] -> w377
                tunnel: w381 -> [_ w400]
                tunnel: w376 -> [_ w396]
                frame False {
                  w394 = 1
                }
                frame True {
                  w403 = 0.75
                  n100 = Unbundle By Name(w396) -> ("Output Element.Total Delay (ms)"=w397:dbl)
                  n101 = Unbundle By Name(w400) -> ("A/D info.# lines per scan"=w398:u16)
                  n102 = Reciprocal(x=w398) -> (1/x=w404:dbl)
                  n103 = Multiply(x=w403, y=w404) -> (x*y=w401:dbl)
                  n104 = Multiply(x=w397, y=w403) -> (x*y=w402:dbl)
                }
              }
              n105 = case shown="False" "Hawk Noise" {
                tunnel: w366 -> [w391 w393]
                tunnel: [w391 w392] -> w367
                frame False {
                }
                frame True {
                  n106 = call "RemNoiseRec.vi"("Data In"=w393) -> ("Data Out"=w392:i16[][])  [unwired: 1 in, 1 out]
                }
              }
              n107 = local write "Keep"(w382) -> ()
              n108 = call "SubMean.vi"("Scan Data In"=w367, "Type of Mean"="Type of Mean") -> ("Array"=w359:dbl[][])  [unwired: 4 in, 2 out]
              n109 = case shown="\"Log Grey Scale\"" "Display mode" {
                tunnel: [w383 w387 w388 w389] -> w358
                tunnel: w359 -> [w384 w386 w388 w390]
                tunnel: w357 -> [_ w385 _ _]
                frame "Linear Abs Grey", Default {
                  n110 = Absolute Value(x=w384) -> (abs(x)=w383:dbl[][])
                }
                frame "Log Grey Scale" {
                  n111 = call "LogScaleImage.vi"("A/D bits"=w385, "input array"=w386) -> ("log scale image"=w387:dbl[][])  [unwired: 1 out]
                }
                frame "Linear Color Scale" {
                }
                frame "dB Scale" {
                  n112 = call "dBScale.vi"("Data In"=w390) -> ("Data Out"=w389:dbl[][])  [unwired: 4 in]
                }
              }
              n113 = call "SetScale.vi"("# A/D bits"=w357, "Display mode"="Display mode") -> ("Array"=w355:cluster{dbl, u32}[])
              n114 = property on="Raw data" class="IntGraph (strict)"("Y Scale.Offset and Multiplier:Offset"=w379, "Y Scale.Offset and Multiplier:Multiplier"=w378, "X Scale.Offset and Multiplier:Multiplier"=w377) -> ()  [unwired: 2 in, 2 out]
              n115 = property on="Raw data" class="IntGraph (strict)"("ZScale.MarkerVals[]"=w355) -> ()  [unwired: 2 in, 2 out]
              n116 = Transpose 2D Array(2D array=w358) -> (transposed array=→"Raw data":dbl[][])
            }
            event "Show Thumbs": Value Change {
              n117 = event-data() -> ()  [unwired: 2 out]
              n118 = Unbundle By Name(w409) -> ("Thumb Size.pixels in x"=w408:i16, "Thumb Size.pixels in y"=w407:i16)
              n119 = call "ShowThumbs.vi"("pixels in y"=w407, "pixels in x"=w408, "columns in display"=3, "Thumbnails In"=w413) -> ()  [unwired: 3 out]
            }
            event "Erase data": Value Change {
              n120 = event-data() -> ()  [unwired: 2 out]
              n121 = Two Button Dialog(message="Warning! Data not saved to disk will be cleared from memory if Erase is selected.", 1:"Return", 2:"Erase") -> (T button?=w435:bool)
              n122 = case shown="False" w435 {
                tunnel: [w447 _] -> w423
                tunnel: [w446 w450] -> w425
                tunnel: [w445 w449] -> w426
                tunnel: w432 -> [w447 _]
                tunnel: w430 -> [w446 _]
                tunnel: w429 -> [w445 _]
                tunnel: w428 -> [w444 _]
                tunnel: [w444 w449] -> w427
                tunnel: [w443 _] -> w424
                tunnel: w431 -> [w443 _]
                tunnel: [w442 _] -> w421
                tunnel: w434 -> [w442 _]
                tunnel: [w441 _] -> w422
                tunnel: w433 -> [w441 _]
                tunnel: [w440 _] -> w420
                tunnel: w419 -> [w440 _]
                frame False {
                }
                frame True {
                  w449 = 0
                  w450 = string[] [] ("Array Constant")
                  # "Erase All Data"
                  n123 = local write "Raw data"(dbl[][] [] ("Raw data")) -> ()
                  n124 = property on="Scan to View" class="Ring (strict)"("Value (Signaling)"=w449) -> ()  [unwired: 2 in, 2 out]
                  n125 = property on="Case\nto View" class="Ring (strict)"("Strings []"=w450) -> ()  [unwired: 2 in, 2 out]
                }
              }
            }
            event "ExitSendCmd": Value Change {
              n126 = event-data() -> ()  [unwired: 2 out]
              n127 = case shown="False" FALSE {
                tunnel: [_ w462] -> w460
                tunnel: w458 -> [_ w461]
                frame False {
                }
                frame True {
                  n128 = call "QuitMode.vi"("hide ftp and quit?"=w461) -> ("mode"=w462:i32)  [unwired: 2 out]
                }
              }
              n129 = case shown="1" w460 {
                tunnel: [TRUE TRUE FALSE] -> w456
                tunnel: w457 -> [_ _ _]
                tunnel: w459 -> [_ _ _]
                frame 0, Default {
                }
                frame 1 {
                  # "Place FTP Data VI\nhere if needed"
                }
                frame 2 {
                }
              }
              n130 = local write "Raw data"(dbl[][] [] ("Raw data")) -> ()
              n131 = property on="Scan to View" class="Ring (strict)"("Strings []"=string[] [] ("Array Constant")) -> ()  [unwired: 2 in, 2 out]
              n132 = property on="Scan to View" class="Ring (strict)"("Val(Sgnl)"=0) -> ()  [unwired: 2 in, 2 out]
            }
            event "Attenuation": Value Change {
              n133 = event-data() -> ("NewVal"=w477:u8)  [unwired: 1 out]
              n134 = case shown="True" TRUE {
                tunnel: w477 -> [_ w478]
                frame False {
                }
                frame True {
                  n135 = call "SetAtt.vi"("Arm Trigs?"=FALSE ("Vecchio Hitachi?"), "Attenuation"=w478) -> ()  [unwired: 1 in, 3 out]
                }
              }
            }
          }
          n136 = Or(x=w133, y=w132) -> (x .or. y?=w139:bool)
        }
      }
      frame #2 {
        # "Stop counter if using B&K 3535"
        n137 = case shown="\"B&K 3535\"" w481 {
          tunnel: w480 -> [_ w482]
          frame "Hitachi", Default {
          }
          frame "B&K 3535" {
            n138 = call <vilib>:"DAQmx Stop Task.vi"("task/channels in"=w482) -> ()  [unwired: 1 in, 14 out]
          }
        }
      }
    }
  }
  "Digitizer Settings" <- w1
  n139 = Unbundle By Name(w1) -> ("Digitizer ID Cluster.GaGe Handle"=w2:T7)
  n140 = case shown="4" w7 {
    tunnel: [TRUE TRUE TRUE TRUE FALSE] -> w6
    frame 0, Default {
    }
    frame 1 {
    }
    frame 2 {
    }
    frame 3 {
    }
    frame 4 {
    }
  }
  n141 = Quit LabVIEW(quit? (T)=w6) -> ()
  n142 = call <userlib>:"CsTool-FreeSystem.vi"("Handle Cluster"=w2) -> ()  [unwired: 1 out]
